vi "Create Plugin Configuration.vi"(6 "plugin timing":T3={"priority"=0, "decimation"=1, "offset"=0}, 8 "channel count per transfer":i32, 9 "transfer configs":T2(array[cluster]), 10 "group configs":cluster{"direction":T4, "timing":T3}[](array[cluster]), 11 "plugin class":string) -> (3 "plugin configuration":T5)   [LabVIEW 2017]
uses:
  Source/Shared/Typedefs/DSF Plugin Configuration.ctl
  Source/DSF Configuration API/1.0.0/Public/Controls/DSF Timing Info.ctl
  Source/Shared/Typedefs/DSF Transfer Group Configuration.ctl
  Source/DSF Configuration API/1.0.0/Public/Controls/DSF Direction.ctl
  Source/Shared/Typedefs/DSF Transfer Configuration.ctl
  Source/DSF Configuration API/1.0.0/Public/Controls/DSF Byte Order.ctl
  Source/Shared/Typedefs/DSF Channel Configuration.ctl
  Source/DSF Configuration API/1.0.0/Public/Controls/DSF Data Type.ctl
  Source/DSF Configuration API/1.0.0/Public/Controls/DSF Settings Info.ctl
  Source/DSF.Engine.lvlib
  Source/DSF Configuration API/1.0.0/DSF Configuration API.lvlib
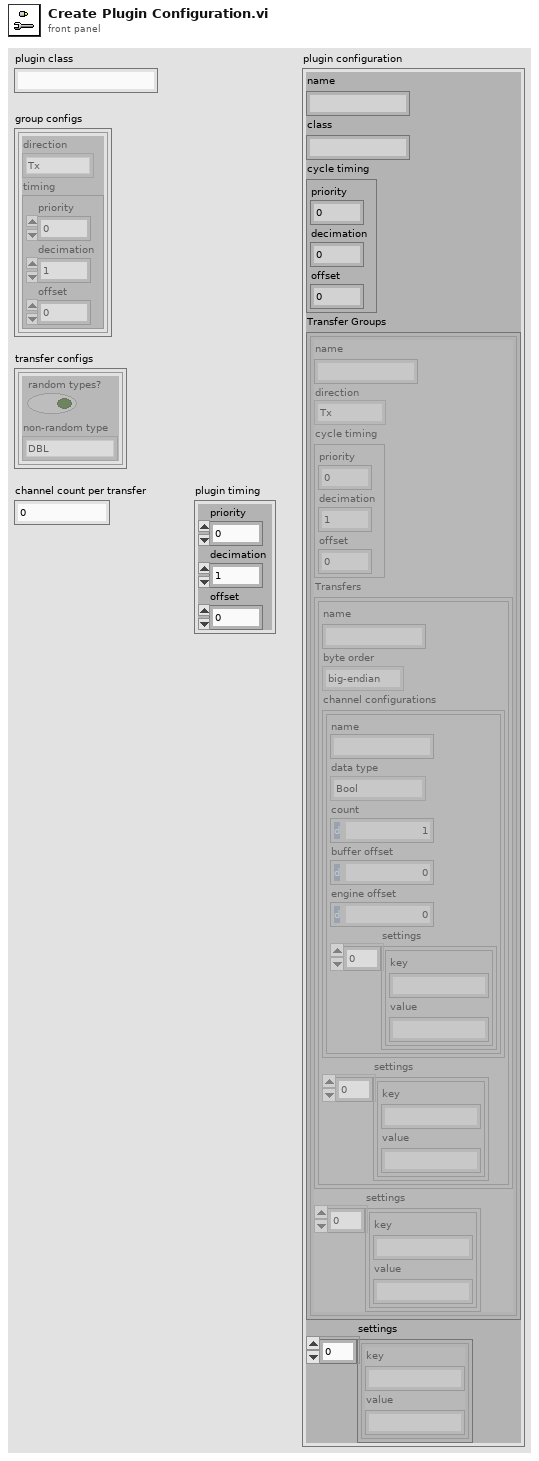
[diagram p1: front panel]
types:
  T1 = typedef "DSF Configuration API.lvlib/DSF Data Type.ctl" = enum8{"Bool", "SGL", "DBL", "I8", "I16", "I32", "I64", "U8", "U16", "U32", "U64"}
  T2 = cluster{"random types?":bool, "non-random type":T1}[]
  T3 = typedef "DSF Configuration API.lvlib/DSF Timing Info.ctl" = cluster{"priority":i32, "decimation":i32, "offset":i32}
  T4 = typedef "DSF Configuration API.lvlib/DSF Direction.ctl" = enum8{"Tx", "Rx"}
  T5 = typedef "DSF.Engine.lvlib/DSF Plugin Configuration.ctl" = cluster{"name":string, "class":string, "cycle timing":T3, "Transfer Groups":T6[], "settings":T10}
  T6 = typedef "DSF.Engine.lvlib/DSF Transfer Group Configuration.ctl" = cluster{"name":string, "direction":T4, "cycle timing":T3, "Transfers":T7[], "settings":T10}
  T7 = typedef "DSF.Engine.lvlib/DSF Transfer Configuration.ctl" = cluster{"name":string, "byte order":T8, "channel configurations":T9[], "settings":T10}
  T8 = typedef "DSF Configuration API.lvlib/DSF Byte Order.ctl" = enum8{"big-endian", "little-endian"}
  T9 = typedef "DSF.Engine.lvlib/DSF Channel Configuration.ctl" = cluster{"name":string, "data type":T1, "count":u64, "buffer offset":u64, "engine offset":u64, "settings":T10}
  T10 = typedef "DSF Configuration API.lvlib/DSF Settings Info.ctl" = cluster{"key":string, "value":string}[]
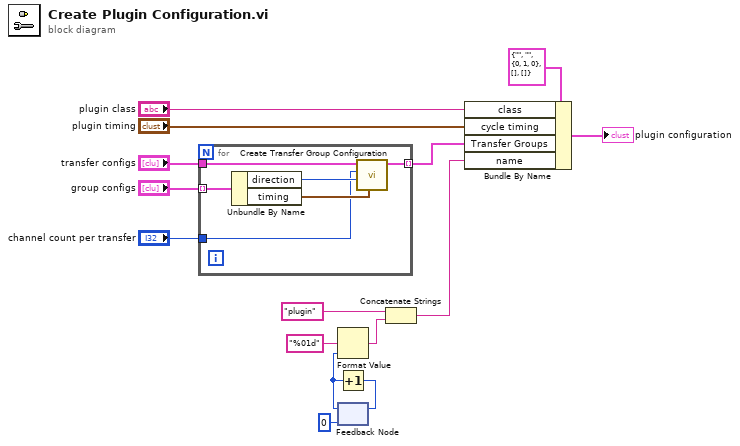
[diagram p0: block diagram]
diagram:
  n1 = for {
    tunnel: [w21] -> w8 mode=indexing
    tunnel: "group configs" -> [w18] mode=indexing
    tunnel: "channel count per transfer" -> [w17]
    tunnel: "transfer configs" -> [w16]
    n2 = Unbundle By Name(w18) -> ("direction"=w20:T4, "timing"=w19:T3)
    n3 = call "Create Transfer Group Configuration.vi"("group timing (dec:1, off: 0)"=w19, "direction"=w20, "channel count per transfer"=w17, "transfer configs"=w16) -> ("transfer group"=w21:T6)  [unwired: 7 in]
  }
  n4 = feedback #1(0) -> (w13:i32)
  n5 = Format Value(format string="%01d", value (0)=w13) -> (output string=w10:string)  [unwired: 1 in]
  n6 = Increment(x=w13) -> (x+1=w14:i32)
  n7 = feedback-in #1(w14) -> ()
  n8 = Concatenate Strings("plugin" ("name"), w10) -> (w5:string)
  n9 = Bundle By Name(cluster=T5 {"name"="", "class"="", "cycle timing"={"priority"=0, "decimation"=1, "offset"=0}, "Transfer Groups"=[], "settings"=[]} ("Plugin Configuration"), "class"="plugin class", "cycle timing"="plugin timing", "Transfer Groups"=w8, "name"=w5) -> (→"plugin configuration":T5)
